vi "Support Display Data.vi"(6 "Pilot Rate (BTU/hr)":dbl=600.0, 7 "FVIR?":bool, 8 "error in (no error)":errorcluster, 11 "All Data Input":T1 {"PLC Data"."PLC Data - LDO"."Timing"."Absolute Time" format="%<%H:%M:%S%3u>t"; "PLC Data"."PLC Data - LDO"."Timing"."Display Time" format="%#.20f"; "PLC Data"."PLC Data - LDO"."Timing"."Test Time Ref" format="%#.20f"; "PLC Data"."PLC Data - LDO"."Timing"."Precondition Time Ref" format="%#.20f"; "PLC Data"."PLC Data - LDO"."Timing"."First Call Time Ref" format="%#.20f"; "PLC Data"."PLC Data - FVIR"."Timing"."Absolute Time" format="%<%H:%M:%S%3u>t"; "PLC Data"."PLC Data - FVIR"."Timing"."Display Time" format="%#.20f"; "PLC Data"."PLC Data - FVIR"."Timing"."Test Time Ref" format="%#.20f"; "PLC Data"."PLC Data - FVIR"."Timing"."Precondition Time Ref" format="%#.20f"; "PLC Data"."PLC Data - FVIR"."Timing"."First Call Time Ref" format="%#.20f"}) -> (0 "error out":errorcluster, 3 "All Data Output":T1 {"PLC Data"."PLC Data - LDO"."Timing"."Absolute Time" format="%<%H:%M:%S%3u>t"; "PLC Data"."PLC Data - LDO"."Timing"."Display Time" format="%#.20f"; "PLC Data"."PLC Data - LDO"."Timing"."Test Time Ref" format="%#.20f"; "PLC Data"."PLC Data - LDO"."Timing"."Precondition Time Ref" format="%#.20f"; "PLC Data"."PLC Data - LDO"."Timing"."First Call Time Ref" format="%#.20f"; "PLC Data"."PLC Data - FVIR"."Timing"."Absolute Time" format="%<%H:%M:%S%3u>t"; "PLC Data"."PLC Data - FVIR"."Timing"."Display Time" format="%#.20f"; "PLC Data"."PLC Data - FVIR"."Timing"."Test Time Ref" format="%#.20f"; "PLC Data"."PLC Data - FVIR"."Timing"."Precondition Time Ref" format="%#.20f"; "PLC Data"."PLC Data - FVIR"."Timing"."First Call Time Ref" format="%#.20f"}, 5 "Burner ON?":bool)   [LabVIEW 2020]
uses:
  Modbus/Modbus All Data.ctl
  Modbus/Modbus PLC Data All.ctl
  Modbus/Modbus FVIR Control.ctl
  Modbus/Modbus Timing.ctl
  <vilib>/Utility/miscctls.llb/LVDateTimeRec.ctl
  Modbus/Modbus LDO Control.ctl
  WritingDataFile/Data to Save.ctl
  Terminate Conditions Cluster.ctl
  Drivers/Inficon Transmitter/Type Definitions/Inficon Data.ctl
  Modbus/Modbus Gas Meter Data.ctl
  Drivers/Alicat LabVIEW Drivers 2v1/Sub-VIs/Data Cluster.ctl
  Drivers/Alicat LabVIEW Drivers 2v1/Sub-VIs/Units of Measure.ctl
  Gas_Rate/HEWH ANSI Rate.ctl
  Drivers/Resideo Gas Valve/Type Definitions/Vesta Info.ctl
  Agilent Data.ctl
panel:
  # "Totalizer Timer"
  # "Totalizer Timer"
  # "Natural Gas"
  # "Propane"
  # "Totalizer Timer"
  # "Totalizer Timer"
  # "Natural Gas"
  # "Propane"
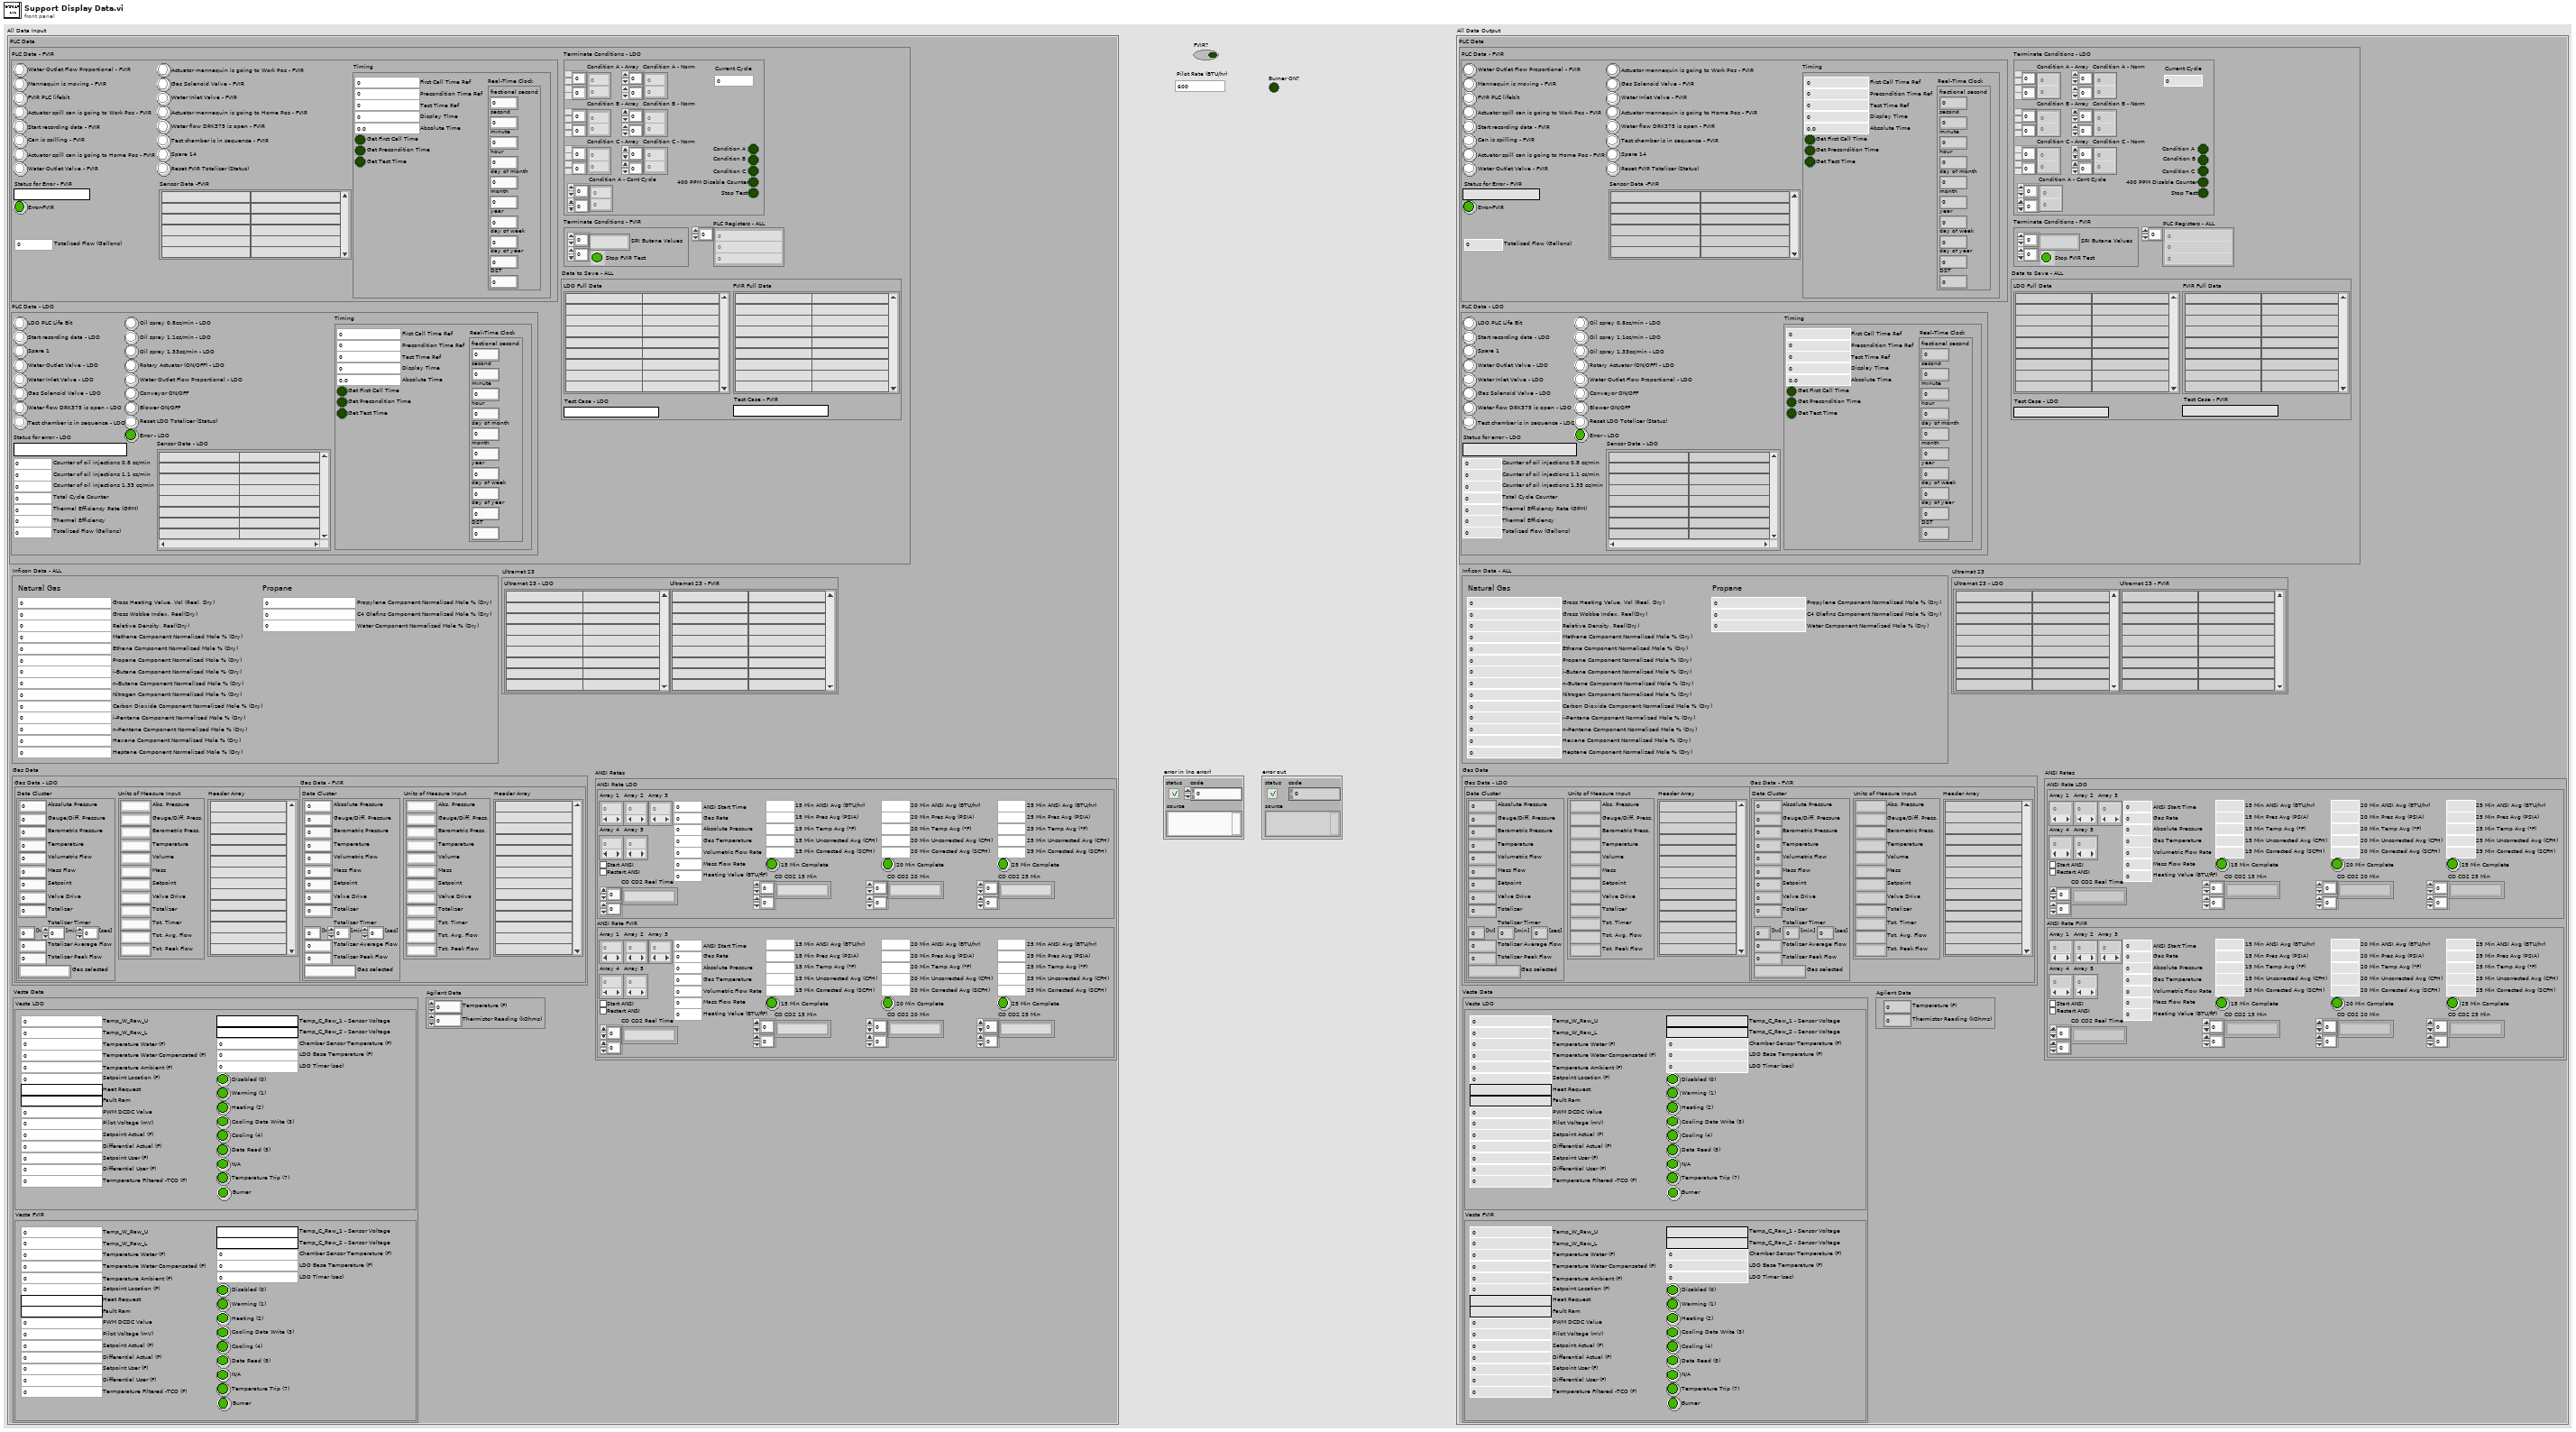
[diagram p1: front panel]
types:
  T1 = typedef "Modbus All Data.ctl" = cluster{"PLC Data":T2, "Inficon Data - ALL":T9, "Gas Data":cluster{"Gas Data - LDO":T10, "Gas Data - FVIR":T10}, "Ultramat 23":cluster{"Ultramat 23 - LDO":string[][], "Ultramat 23 - FVIR":string[][]}, "ANSI Rates":cluster{"ANSI Rate LDO":T13, "ANSI Rate FVIR":T13}, "Vesta Data":cluster{"Vesta LDO":T14, "Vesta FVIR":T14}, "Agilent Data":T15}
  T2 = typedef "Modbus PLC Data All.ctl" = cluster{"PLC Data - FVIR":T3, "PLC Data - LDO":T6, "PLC Registers - ALL":i16[], "Data to Save - ALL":T7, "Terminate Conditions - LDO":T8, "Terminate Conditions - FVIR":cluster{"SRI Butane Values":string[][], "Stop FVIR Test":bool}}
  T3 = typedef "Modbus FVIR Control.ctl" = cluster{"Reset FVIR Totalizer (Status)":bool, "Spare 14":bool, "Actuator mannequin is going to Work Pos - FVIR":bool, "Actuator mannequin is going to Home Pos - FVIR":bool, "Test chamber is in sequence - FVIR ":bool, "Water flow DRK375 is open - FVIR":bool, "Gas Solenoid Valve - FVIR":bool, "Water Inlet Valve - FVIR":bool, "Water Outlet Flow Proportional - FVIR":bool, "Start recording data - FVIR":bool, "Actuator spill can is going to Work Pos - FVIR":bool, "Actuator spill can is going to Home Pos - FVIR":bool, "Water Outlet Valve - FVIR":bool, "Can is spilling - FVIR":bool, "Mannequin is moving - FVIR":bool, "FVIR PLC lifebit":bool, "Status for Error - FVIR":string, "Error-FVIR":bool, "Sensor Data -FVIR":string[][], "Totalized Flow (Gallons)":dbl, "Timing":T4}
  T4 = typedef "Modbus Timing.ctl" = cluster{"First Call Time Ref":dbl, "Precondition Time Ref":dbl, "Test Time Ref":dbl, "Get First Call Time":bool, "Get Precondition Time":bool, "Get Test Time":bool, "Display Time":dbl, "Real-Time Clock":T5, "Absolute Time":dbl}
  T5 = typedef "LVDateTimeRec.ctl" = cluster{"fractional second":dbl, "second":i32, "minute":i32, "hour":i32, "day of month":i32, "month":i32, "year":i32, "day of week":i32, "day of year":i32, "DST":i32}
  T6 = typedef "Modbus LDO Control.ctl" = cluster{"LDO PLC Life Bit":bool, "Start recording data - LDO":bool, "Spare 1":bool, "Water Outlet Valve - LDO":bool, "Water Inlet Valve - LDO":bool, "Gas Solenoid Valve - LDO":bool, "Water flow DRK375 is open - LDO":bool, "Test chamber is in sequence - LDO":bool, "Oil spray 0.8cc/min - LDO":bool, "Oil spray 1.1cc/min - LDO":bool, "Oil spray 1.33cc/min - LDO":bool, "Rotary Actuator (ON/OFF) - LDO":bool, "Water Outlet Flow Proportional - LDO":bool, "Conveyor ON/OFF":bool, "Blower ON/OFF":bool, "Reset LDO Totalizer (Status)":bool, "Status for error - LDO":string, "Error - LDO":bool, "Sensor Data - LDO":string[][], "Thermal Efficiency Rate (GPM)":dbl, "Thermal Efficiency":dbl, "Totalized Flow (Gallons)":dbl, "Counter of oil injections 1.33 cc/min":u16, "Total Cycle Counter":u16, "Counter of oil injections 1.1 cc/min":u16, "Counter of oil injections 0.8 cc/min":u16, "Timing":T4}
  T7 = typedef "Data to Save.ctl" = cluster{"LDO Full Data":string[][], "FVIR Full Data":string[][], "Test Case - FVIR":string, "Test Case - LDO":string}
  T8 = typedef "Terminate Conditions Cluster.ctl" = cluster{"Condition B - Array":dbl[][], "Current Cycle":u16, "Condition C - Array":dbl[][], "Condition A - Array":dbl[][], "400 PPM Disable Counter":bool, "Condition A - Norm":dbl[][], "Condition B - Norm":dbl[][], "Condition C - Norm":dbl[][], "Condition A":bool, "Condition B":bool, "Condition C":bool, "Condition A - Cont Cycle":dbl[][], "Stop Test":bool}
  T9 = typedef "Inficon Data.ctl" = cluster{"Gross Heating Value, Vol (Real, Dry)":dbl, "Nitrogen Component Normalized Mole % (Dry)":dbl, "Methane Component Normalized Mole % (Dry)":dbl, "Carbon Dioxide Component Normalized Mole % (Dry)":dbl, "Ethane Component Normalized Mole % (Dry)":dbl, "Propane Component Normalized Mole % (Dry)":dbl, "i-Pentane Component Normalized Mole % (Dry)":dbl, "i-Butane Component Normalized Mole % (Dry)":dbl, "n-Butane Component Normalized Mole % (Dry)":dbl, "n-Pentane Component Normalized Mole % (Dry)":dbl, "Hexane Component Normalized Mole % (Dry)":dbl, "Heptane Component Normalized Mole % (Dry)":dbl, "Gross Wobbe Index, Real(Dry)":dbl, "Relative Density, Real(Dry)":dbl, "Propylene Component Normalized Mole % (Dry)":dbl, "C4 Olefins Component Normalized Mole % (Dry)":dbl, "Water Component Normalized Mole % (Dry)":dbl}
  T10 = typedef "Modbus Gas Meter Data.ctl" = cluster{"Data Cluster":T11, "Units of Measure Input":T12, "Header Array":string[]}
  T11 = typedef "Data Cluster.ctl" = cluster{"Absolute Pressure":dbl, "Gauge/Diff. Pressure":dbl, "Barometric Pressure":dbl, "Temperature":dbl, "Volumetric Flow":dbl, "Mass Flow":dbl, "Setpoint":dbl, "Valve Drive":dbl, "Totalizer":dbl, "[hr]":dbl, "[min]":dbl, "[sec]":dbl, "Totalizer Average Flow":dbl, "Totalizer Peak Flow":dbl, "Gas selected":string}
  T12 = typedef "Units of Measure.ctl" = cluster{"Abs. Pressure":string, "Gauge/Diff. Press.":string, "Barometric Press.":string, "Temperature":string, "Volume":string, "Mass":string, "Setpoint":string, "Valve Drive":string, "Totalizer":string, "Tot. Timer":string, "Tot. Avg. Flow":string, "Tot. Peak Flow":string}
  T13 = typedef "HEWH ANSI Rate.ctl" = cluster{"Array 1":dbl[], "Array 3":dbl[], "Array 2":dbl[], "Start ANSI":bool, "ANSI Start Time":dbl, "Restart ANSI":bool, "15 Min ANSI Avg (BTU/hr)":dbl, "20 Min ANSI Avg (BTU/hr)":dbl, "25 Min ANSI Avg (BTU/hr)":dbl, "Absolute Pressure":dbl, "Gas Temperature":dbl, "Volumetric Flow Rate":dbl, "Mass Flow Rate":dbl, "Array 4":dbl[], "Array 5":dbl[], "Gas Rate":dbl, "15 Min Pres Avg (PSIA)":dbl, "20 Min Pres Avg (PSIA)":dbl, "25 Min Pres Avg (PSIA)":dbl, "15 Min Temp Avg (°F) ":dbl, "20 Min Temp Avg (°F)":dbl, "25 Min Temp Avg (°F)":dbl, "15 Min Uncorrected Avg (CFH)":dbl, "20 Min Uncorrected Avg (CFH)":dbl, "25 Min Uncorrected Avg (CFH)":dbl, "15 Min Corrected Avg (SCFH)":dbl, "20 Min Corrected Avg (SCFH)":dbl, "25 Min Corrected Avg (SCFH)":dbl, "15 Min Complete":bool, "20 Min Complete":bool, "25 Min Complete":bool, "Heating Value (BTU/ft³)":dbl, "CO CO2 15 Min":string[][], "CO CO2 20 Min":string[][], "CO CO2 25 Min":string[][], "CO CO2 Real Time":string[][]}
  T14 = typedef "Vesta Info.ctl" = cluster{"Temp_W_Raw_U":u16, "Temp_W_Raw_L":u16, "Temperature Water (F)":dbl, "Temperature Water Compensated (F)":dbl, "Temperature Ambient (F)":dbl, "Setpoint Location (F)":dbl, "Heat Request":string, "Fault Ram":string, "PWM DCDC Value":u16, "Pilot Voltage (mV)":dbl, "Setpoint Actual (F)":dbl, "Differential Actual (F)":dbl, "Setpoint User (F)":dbl, "Differential User (F)":dbl, "Termperature FIltered -TCO (F)":dbl, "Temp_C_Raw_1 - Sensor Voltage":string, "Temp_C_Raw_2 - Sensor Voltage":string, "Chamber Sensor Temperature (F)":dbl, "LDO Base Temperature (F)":dbl, "LDO Timer (sec)":i16, "Disabled (0)":bool, "Warming (1)":bool, "Heating (2)":bool, "Cooling Data Write (3)":bool, "Cooling (4)":bool, "Data Read (5)":bool, "N/A":bool, "Temperature Trip (7)":bool, "Burner":bool}
  T15 = typedef "Agilent Data.ctl" = cluster{"Temperature (F)":dbl, "Thermistor Reading (kOhms)":dbl}
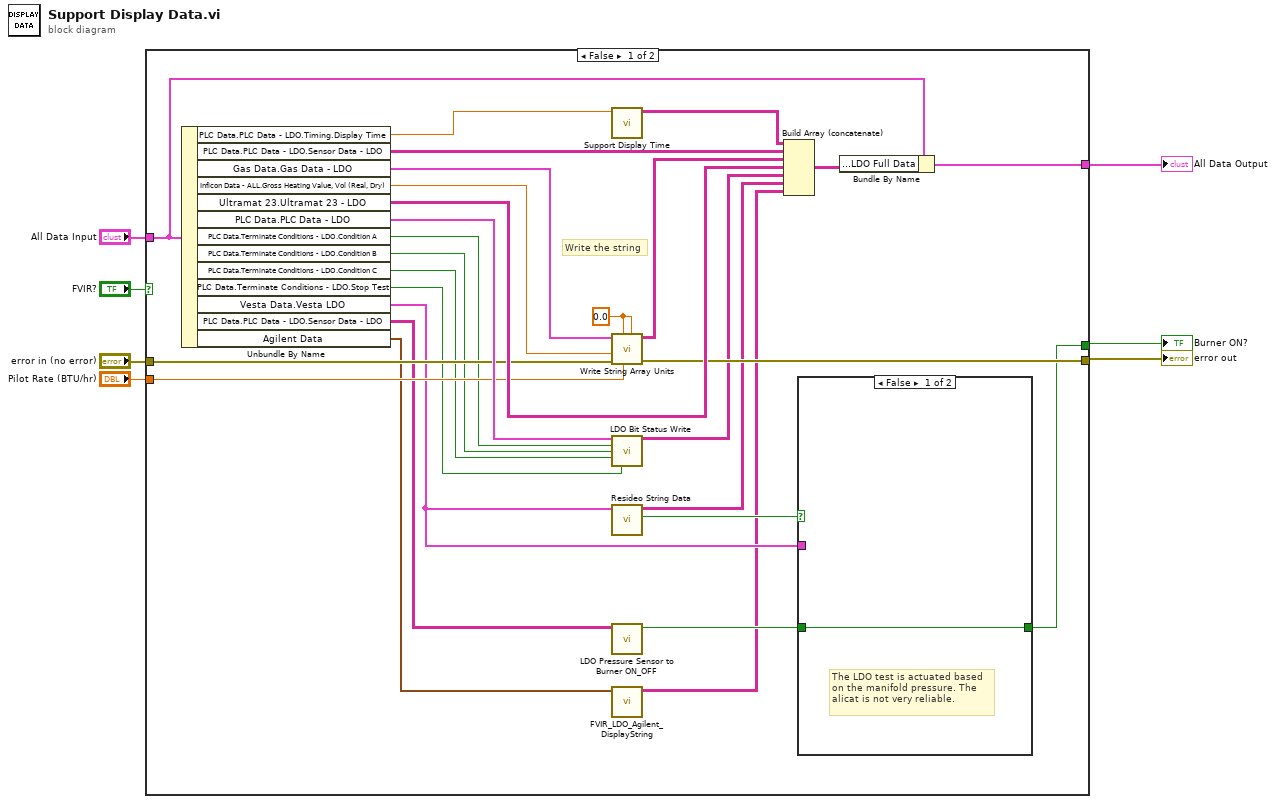
[diagram p0: block diagram]
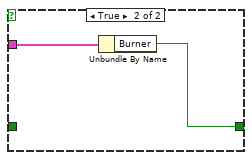
[diagram p2: hidden frame]
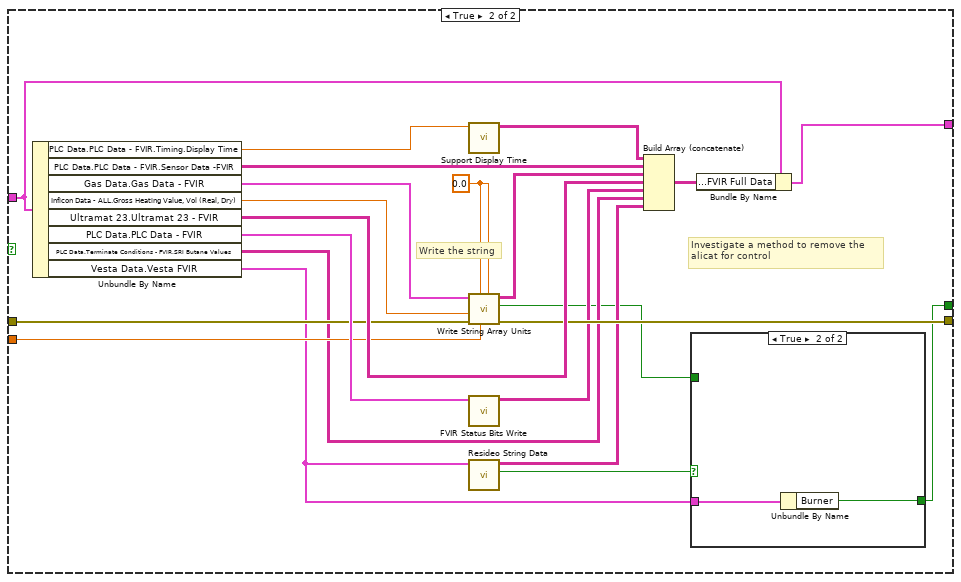
[diagram p3: hidden frame]
diagram:
  n1 = case shown="False" "FVIR?" {
    tunnel: [w28 w49] -> w7
    tunnel: "error in (no error)" -> [w25 w50]
    tunnel: "Pilot Rate (BTU/hr)" -> [w23 w48]
    tunnel: [w12 w40] -> w4
    tunnel: "All Data Input" -> [w22 w47]
    tunnel: [w21 w46] -> w2
    frame False {
      w27 = 0.0 ("HHV_1")
      # "Write the string"
      n2 = Unbundle By Name(w22) -> ("PLC Data.PLC Data - LDO.Timing.Display Time"=w31:dbl, "PLC Data.PLC Data - LDO.Sensor Data - LDO"=w32:string[][], "Gas Data.Gas Data - LDO"=w34:T10, "Inficon Data - ALL.Gross Heating Value, Vol (Real, Dry)"=w30:dbl, "Ultramat 23.Ultramat 23 - LDO"=w33:string[][], "PLC Data.PLC Data - LDO"=w35:T6, "PLC Data.Terminate Conditions - LDO.Condition A"=w19:bool, "PLC Data.Terminate Conditions - LDO.Condition B"=w18:bool, "PLC Data.Terminate Conditions - LDO.Condition C"=w17:bool, "PLC Data.Terminate Conditions - LDO.Stop Test"=w16:bool, "Vesta Data.Vesta LDO"=w14:T14, "PLC Data.PLC Data - LDO.Sensor Data - LDO"=w11:string[][], "Agilent Data"=w9:T15)
      n3 = call "Support Display Time.vi"("Display Time"=w31) -> ("Total Array"=w29:string[][])  [unwired: 10 in]
      n4 = call "Write String Array Units.vi"("Total_1"=w27, "Pilot Rate (BTU/hr)"=w23, "HHV_1"=w27, "Error In"=w25, "Gross Heating Value, Vol (Real, Dry)"=w30, "Gas Data"=w34) -> ("Error Out"=w28:errorcluster, "String Data"=w26:string[][])  [unwired: 3 in, 1 out]
      n5 = call "LDO Bit Status Write.vi"("LDO Control Input"=w35, "Condition A"=w19, "Condition B"=w18, "Condition C"=w17, "Stop Test"=w16) -> ("Bit Status"=w24:string[][])  [unwired: 9 in, 1 out]
      n6 = call "Resideo String Data.vi"("Vesta LDO"=w14) -> ("Trigger Vesta Burner Control"=w13:bool, "Vesta Data"=w15:string[][])  [unwired: 8 in, 1 out]
      n7 = call "LDO Pressure Sensor to Burner ON_OFF.vi"("Sensor Data - LDO"=w11) -> ("Burner ON?"=w10:bool)  [unwired: 9 in, 1 out]
      n8 = call "FVIR_LDO_Agilent_DisplayString.vi"("Agilent Data in"=w9) -> ("transposed array"=w8:string[][])  [unwired: 10 in]
      n9 = Build Array (concatenate)(w29, w32, w26, w33, w24, w15, w8) -> (w20:string[][])
      n10 = case shown="False" w13 {
        tunnel: w10 -> [w36 _]
        tunnel: [w36 w37] -> w12
        tunnel: w14 -> [_ w38]
        frame False {
          # "The LDO test is actuated based\non the manifold pressure. The \nalicat is not very reliable."
        }
        frame True {
          n11 = Unbundle By Name(w38) -> ("Burner"=w37:bool)
        }
      }
      n12 = Bundle By Name(cluster=w22, "PLC Data.Data to Save - ALL.LDO Full Data"=w20) -> (w21:T1)
    }
    frame True {
      w57 = 0.0 ("HHV_1")
      # "Investigate a method to remove the \nalicat for control"
      # "Write the string"
      n13 = Unbundle By Name(w47) -> ("PLC Data.PLC Data - FVIR.Timing.Display Time"=w56:dbl, "PLC Data.PLC Data - FVIR.Sensor Data -FVIR"=w55:string[][], "Gas Data.Gas Data - FVIR"=w54:T10, "Inficon Data - ALL.Gross Heating Value, Vol (Real, Dry)"=w53:dbl, "Ultramat 23.Ultramat 23 - FVIR"=w52:string[][], "PLC Data.PLC Data - FVIR"=w51:T3, "PLC Data.Terminate Conditions - FVIR.SRI Butane Values"=w44:string[][], "Vesta Data.Vesta FVIR"=w39:T14)
      n14 = call "Support Display Time.vi"("Display Time"=w56) -> ("Total Array"=w60:string[][])  [unwired: 10 in]
      n15 = call "Write String Array Units.vi"("Total_1"=w57, "Pilot Rate (BTU/hr)"=w48, "HHV_1"=w57, "Error In"=w50, "Gross Heating Value, Vol (Real, Dry)"=w53, "Gas Data"=w54) -> ("Error Out"=w49:errorcluster, "Burner ON?"=w41:bool, "String Data"=w59:string[][])  [unwired: 3 in]
      n16 = call "FVIR Status Bits Write.vi"("PLC Data - FVIR Input"=w51) -> ("Bit Status"=w45:string[][])  [unwired: 10 in]
      n17 = call "Resideo String Data.vi"("Vesta LDO"=w39) -> ("Trigger Vesta Burner Control"=w42:bool, "Vesta Data"=w43:string[][])  [unwired: 8 in, 1 out]
      n18 = Build Array (concatenate)(w60, w55, w59, w52, w45, w44, w43) -> (w58:string[][])
      n19 = case shown="True" w42 {
        tunnel: w41 -> [w61 _]
        tunnel: [w61 w62] -> w40
        tunnel: w39 -> [_ w63]
        frame False {
        }
        frame True {
          n20 = Unbundle By Name(w63) -> ("Burner"=w62:bool)
        }
      }
      n21 = Bundle By Name(cluster=w47, "PLC Data.Data to Save - ALL.FVIR Full Data"=w58) -> (w46:T1)
    }
  }
  "error out" <- w7
  "Burner ON?" <- w4
  "All Data Output" <- w2
